vi "get FPGA resource reservation info.vi"(8 "error in (no error)":errorcluster, 10 "Name in Bitfile":string, 11 "Item Ref in":T1 format="%.0x") -> (0 "error out":errorcluster, 1 "found?":bool, 2 "Reserver Node Ref":T1=18446744073709551615 format="%.0x", 3 "Item Ref out":T1 format="%.0x", 4 "notes":string)   [LabVIEW 2016, in "FPGA RM Client API.lvlib"]
uses:
  FPGA RM Client API.lvlib
  <vilib>/NI Veristand/Custom Device API/Custom Device Item Ref.ctl
  <vilib>/NI VeriStand/Custom Device API/Custom Device API.lvlib
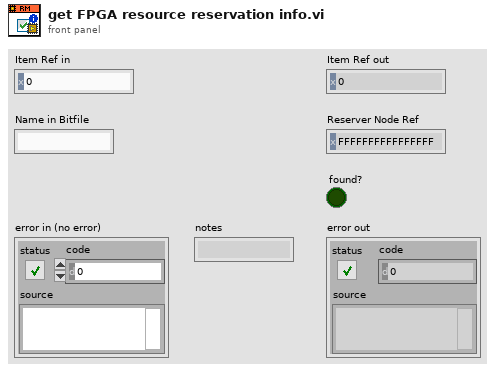
[diagram p1: front panel]
types:
  T1 = typedef "Custom Device API.lvlib/Custom Device Item Ref.ctl" = u64
  T2 = typedef "FPGA RM Client API.lvlib/fpga resource.ctl" = cluster{"name":string, "datatype":string, "channel type":T3, "value":variant, "notes":string}
  T3 = typedef "FPGA RM Client API.lvlib/Channel Type.ctl" = enum16{"Write Channel", "Read Channel", "Write Waveform", "Read Waveform"}
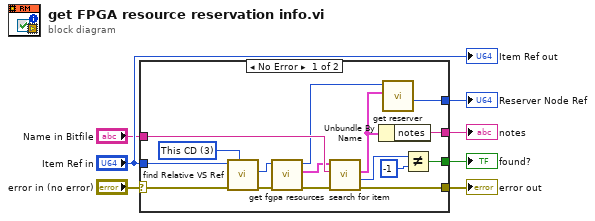
[diagram p0: block diagram]
diagram:
  n1 = case shown="No Error" "error in (no error)" {
    selector: "error in (no error)" -> [w20 w24]
    tunnel: [w14 w24] -> w6
    tunnel: "Item Ref in" -> [w21 _]
    tunnel: "Name in Bitfile" -> [w19 _]
    tunnel: [w16 _] -> w3
    tunnel: [w8 _] -> w2
    tunnel: [w15 _] -> w1
    frame No Error {
      w23 = u16 3 items=["Targets", "Controller", "Custom Devices", "This CD", "This CD/Group", "This CD/Group/SubGroup"] ("Relative Type")
      n2 = call "find Relative VS Ref.vi"("Relative Type"=w23, "error in (no error)"=w20, "Item Ref in"=w21) -> ("error out"=w22:errorcluster, "Relative Item Ref Out"=w12:T1)  [unwired: 4 in, 3 out]
      n3 = call "get fgpa resources.vi"("error in (no error)"=w22, "Item Ref in"=w12) -> ("error out"=w13:errorcluster, "get fpga resources"=w11:T2[], "Item Ref out"=w10:T1)  [unwired: 6 in, 1 out]
      n4 = call "search for item.vi"("error in (no error)"=w13, "Name in bitfile"=w19, "FPGA Resources in"=w11) -> ("error out"=w14:errorcluster, "index of element"=w18:i32, "FPGA Resource"=w9:T2)  [unwired: 6 in]
      n5 = Unbundle By Name(w9) -> ("notes"=w15:string)
      n6 = call "get reserver.vi"("FPGA Resource"=w9, "Item Ref in"=w10) -> ("Dependent Node Ref"=w8:T1)  [unwired: 7 in, 2 out]
      n7 = Not Equal?(x=w18, y=-1) -> (x != y?=w16:bool)
    }
    frame Error {
    }
  }
  "error out" <- w6
  "found?" <- w3
  "Reserver Node Ref" <- w2
  "notes" <- w1
  "Item Ref out" <- "Item Ref in"
